vi "VI.close_fp_lua.vi"(5 "LuaVIEW reference":T1) -> (15 "error out":errorcluster)   [LabVIEW 2012]
doc: "Closes the front panel of a VI. This method maps to the LabVIEW close fp VI method. When the front panel is already closed, no action is under taken.\nParameters:\nobj:self, object of the VI.\nErrors:\nNot a VI object.\nDead VI object.\nCould not close front panel."
uses:
  typedefs/t_LuaVIEW Reference.ctl
  subvis/private/LuaVIEW Pull (object).vi
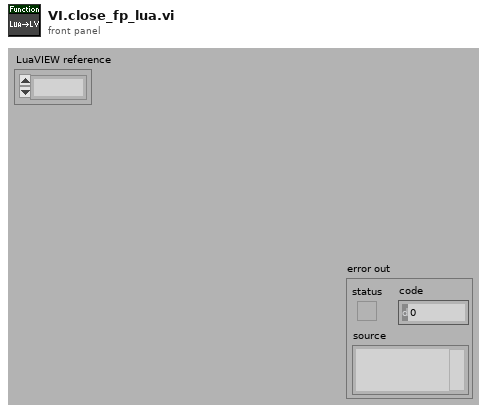
[diagram p1: front panel]
types:
  T1 = typedef "t_LuaVIEW Reference.ctl" = refnum<k1>
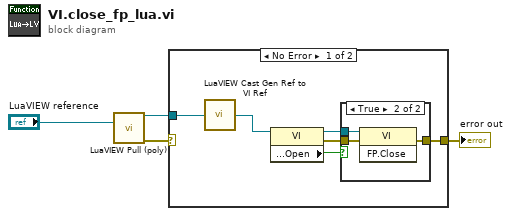
[diagram p0: block diagram]
diagram:
  n1 = call-poly "LuaVIEW Pull (poly).vi"("LuaVIEW reference in"="LuaVIEW reference") -> ("object refnum"=w2:refnum<vi>, "error out"=w1:errorcluster)  [unwired: 11 in, 2 out]
  n2 = case shown="No Error" w1 {
    selector: w1 -> [_ w15]
    tunnel: [w10 w15] -> w3
    tunnel: w2 -> [w9 _]
    frame No Error {
      n3 = call "LuaVIEW Cast Gen Ref to VI Ref.vi"("refnum in"=w9) -> ("refnum out"=w8:refnum<vi>)  [unwired: 14 in]
      n4 = property class="VI"(reference=w8) -> (reference out=w7:refnum<vi>, error out=w6:errorcluster, "Front Panel Window:Open"=w5:bool)  [unwired: 1 in]
      n5 = case shown="True" w5 {
        tunnel: [w11 w14] -> w10
        tunnel: w7 -> [_ w13]
        tunnel: w6 -> [w11 w12]
        frame False {
        }
        frame True {
          n6 = invoke class="VI" method="FP.Close"(reference=w13, error in=w12) -> (error out=w14:errorcluster)  [unwired: 1 in, 2 out]
        }
      }
    }
    frame Error {
    }
  }
  "error out" <- w3
